vi "Error2Txt.vi"(5 "Error in":string) -> (2 "Description out":string)   [LabVIEW 2015, in "Pfeiffer Vacuum.lvlib"]
uses:
  Pfeiffer Vacuum.lvlib
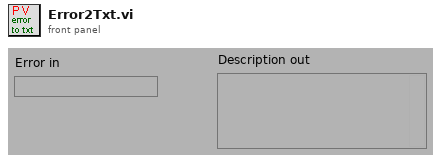
[diagram p1: front panel]
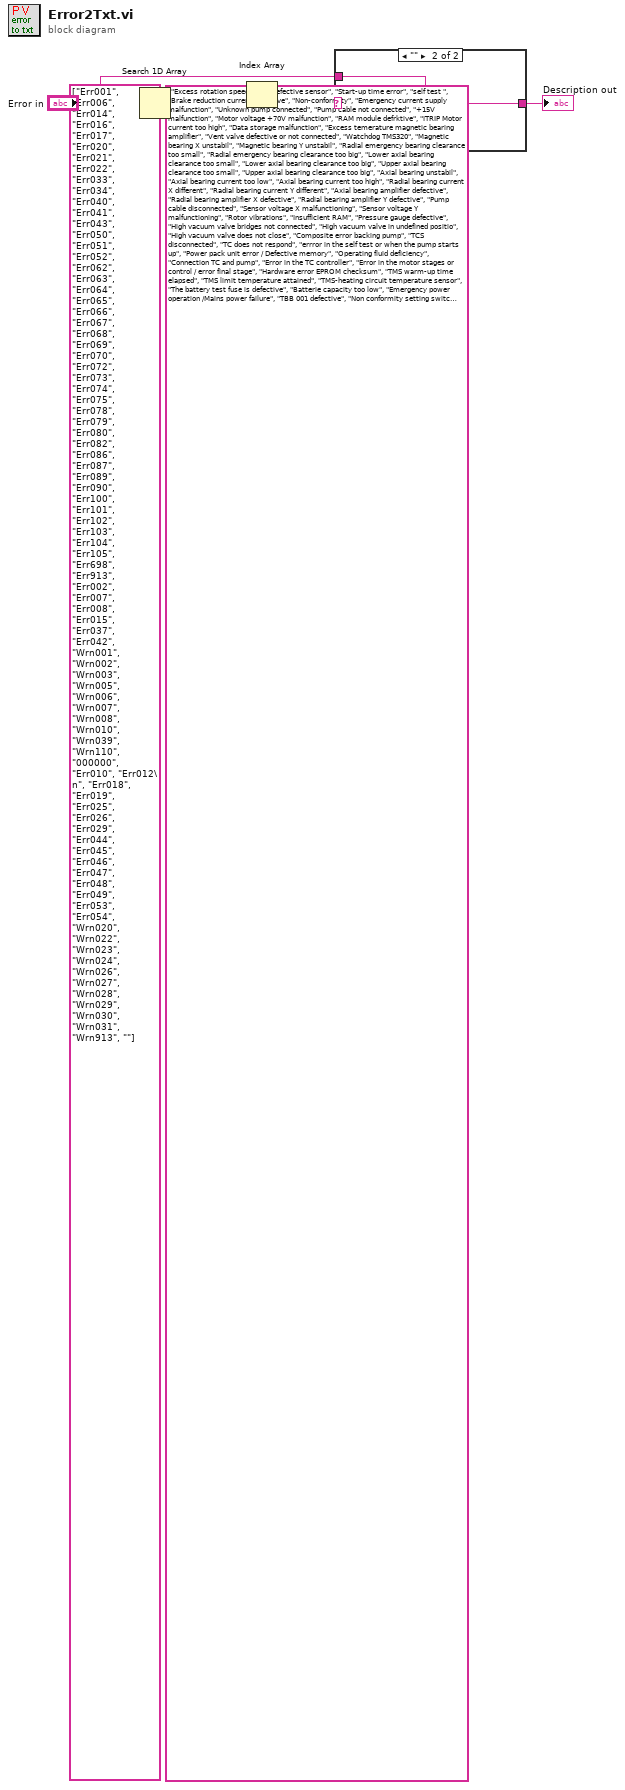
[diagram p0: block diagram]
diagram:
  n1 = Search 1D Array(1D array=string[] ["Err001", "Err006", "Err014", "Err016", "Err017", "Err020", "Err021", "Err022", "Err033", "Err034", "Err040", "Err041", "Err043", "Err050", "Err051", "Err052", "Err062", "Err063", "Err064", "Err065", "Err066", "Err067", "Err068", "Err069", "Err070", "Err072", "Err073", "Err074", "Err075", "Err078", "Err079", "Err080", "Err082", "Err086", "Err087", "Err089", "Err090", "Err100", "Err101", "Err102", "Err103", "Err104", "Err105", "Err698", "Err913", "Err002", "Err007", "Err008", "Err015", "Err037", "Err042", "Wrn001", "Wrn002", "Wrn003", "Wrn005", "Wrn006", "Wrn007", "Wrn008", "Wrn010", "Wrn039", "Wrn110", "000000", "Err010", "Err012\n", "Err018", "Err019", "Err025", "Err026", "Err029", "Err044", "Err045", "Err046", "Err047", "Err048", "Err049", "Err053", "Err054", "Wrn020", "Wrn022", "Wrn023", "Wrn024", "Wrn026", "Wrn027", "Wrn028", "Wrn029", "Wrn030", "Wrn031", "Wrn913", ""] ("1D Array"), element="Error in") -> (index of element=w4:i32)  [unwired: 1 in]
  n2 = Index Array(array=string[] ["Excess rotation speed TMP / Defective sensor", "Start-up time error", "self test ", "Brake reduction current defective", "Non-conformity", "Emergency current supply malfunction", "Unknown pump connected", "Pump cable not connected", "+15V malfunction", "Motor voltage +70V malfunction", "RAM module defrktive", "ITRIP Motor current too high", "Data storage malfunction", "Excess temerature magnetic bearing amplifier", "Vent valve defective or not connected", "Watchdog TMS320", "Magnetic bearing X unstabil", "Magnetic bearing Y unstabil", "Radial emergency bearing clearance too small", "Radial emergency bearing clearance too big", "Lower axial bearing clearance too small", "Lower axial bearing clearance too big", "Upper axial bearing clearance too small", "Upper axial bearing clearance too big", "Axial bearing unstabil", "Axial bearing current too low", "Axial bearing current too high", "Radial bearing current X different", "Radial bearing current Y different", "Axial bearing amplifier defective", "Radial bearing amplifier X defective", "Radial bearing amplifier Y defective", "Pump cable disconnected", "Sensor voltage X malfunctioning", "Sensor voltage Y malfunctioning", "Rotor vibrations", "Insufficient RAM", "Pressure gauge defective", "High vacuum valve bridges not connected", "High vacuum valve in undefined positio", "High vacuum valve does not close", "Composite error backing pump", "TCS disconnected", "TC does not respond", "errror in the self test or when the pump starts up", "Power pack unit error / Defective memory", "Operating fluid deficiency", "Connection TC and pump", "Error in the TC controller", "Error in the motor stages or control / error final stage", "Hardware error EPROM checksum", "TMS warm-up time elapsed", "TMS limit temperature attained", "TMS-heating circuit temperature sensor", "The battery test fuse is defective", "Batterie capacity too low", "Emergency power operation /Mains power failure", "TBB 001 defective", "Non conformity setting switch output", "Protective conductor warning TC", "Pressure gauge defective", "No error", "initialization of driveunit failed", "Inletgauges cross values", "exhaustpressure sensor disconnected", "exhaustpressure to high", "Measurement casetemperature : path interrupted", "Measurement casetemperature : short circuit", "Flowmeter self test failed or Inert gas unit is defective", "Overtemperature electronic", "Overtemperature motor", "E2PROM access error", "timeout selftest", "Intakepressure gauge 1 disconnected", "Intakepressure gauge 2 disconnected", "Measurement gastemperature : path interupted", "Measurement gastemperature : short circuit", "Bypass valve disconnected", "Gasballastvalve disconnected", "Purgegasvalve disconnected", "Sealvalve disconnected", "only inletgauge 2 installed", "Softpumping error", "Softpumping pressure signal failed ", "Exhausttemperature below setpoint", "Exhausttemperature above setpoint", "Exhausttemperature below setpoint  = > above setpoint", "Rotating direction failed", ""] ("1D Array"), index=w4) -> (element=w3:string)
  n3 = case shown="\"\"" w3 {
    selector: w3 -> [w7 _]
    tunnel: [w7 w8] -> w2
    tunnel: "Error in" -> [_ w8]
    frame Default {
    }
    frame "" {
    }
  }
  "Description out" <- w2
